vi "Comms.vi"(1 "Array":dbl[][](array[numeric])) -> (0 "String":string)   [LabVIEW 2012]
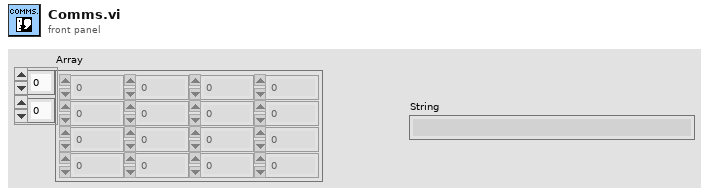
[diagram p1: front panel]
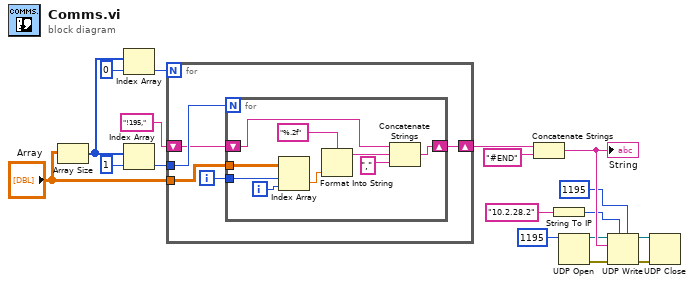
[diagram p0: block diagram]
diagram:
  n1 = Array Size(array="Array") -> (size(s)=w15:i32[])
  n2 = Index Array(array=w15, index=0) -> (element=w17:i32)
  n3 = Index Array(array=w15, index=1) -> (element=w14:i32)
  n4 = for {
    N: w17 -> [_]
    tunnel: w14 -> [w23]
    shift-right: [w21] -> w11
    shift-left: "!195," -> [w22]
    tunnel: "Array" -> [w20]
    i -> [w19]
    n5 = for {
      N: w23 -> [_]
      shift-right: [w31] -> w21
      shift-left: w22 -> [w32]
      tunnel: w20 -> [w29]
      tunnel: w19 -> [w28]
      i -> [w27]
      n6 = Index Array(array=w29, index (row)=w28, index (col)=w27) -> (element=w26:dbl)
      n7 = Format Into String(format string="%.2f", w26) -> (resulting string=w25:string)  [unwired: 2 in, 1 out]
      n8 = Concatenate Strings(w32, w25, "," ("string")) -> (w31:string)
    }
  }
  n9 = Concatenate Strings(w11, "#END" ("string")) -> (w9:string)
  "String" <- w9
  n10 = String To IP(1:"10.2.28.2" ("name")) -> (0:w8:u32)
  n11 = UDP Open(11:u16 1195 ("port")) -> (port=w6:refnum<k16>, 0:w5:errorcluster)  [unwired: 4 in, 1 out]
  n12 = UDP Write(address=w8, port or service name=u16 1195, connection ID=w6, data in=w9, 8:w5) -> (error out=w3:errorcluster, 3:w2:refnum<k16>)  [unwired: 1 in]
  n13 = UDP Close(connection ID=w2, 8:w3) -> ()  [unwired: 2 out]
